vi "LOG_AppendEvent.vi"(8 "error in (no error)":errorcluster, 10 "Log Event":T1, 11 "String in":string) -> (0 "error out":errorcluster, 3 "String out":string)   [LabVIEW 2014]
uses:
  Controls/LOG_MessageQueue.ctl
  <userlib>/_OpenG.lib/string/string.llb/Trim Whitespace (String)__ogtk.vi
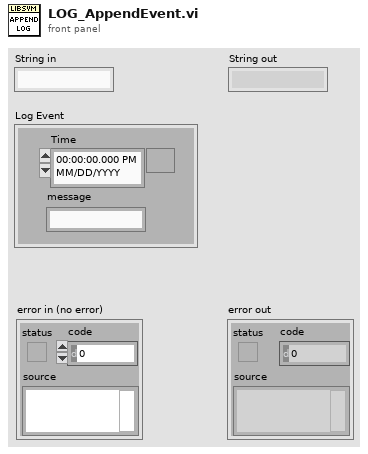
[diagram p1: front panel]
types:
  T1 = typedef "LOG_MessageQueue.ctl" = cluster{"Time":timestamp, "message":string}
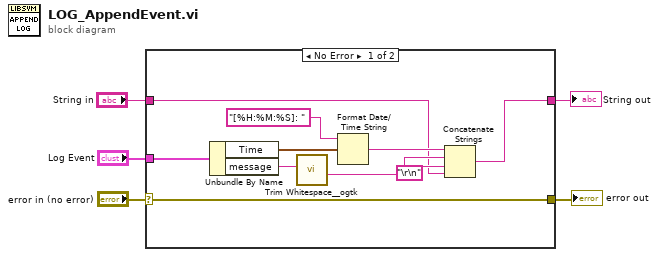
[diagram p0: block diagram]
diagram:
  n1 = case shown="No Error" "error in (no error)" {
    selector: "error in (no error)" -> [w6 w17]
    tunnel: [w6 w17] -> w5
    tunnel: [w9 w16] -> w3
    tunnel: "Log Event" -> [w8 _]
    tunnel: "String in" -> [w7 w16]
    frame No Error {
      n2 = Unbundle By Name(w8) -> ("Time"=w13:timestamp, "message"=w11:string)
      n3 = call-poly <userlib>:"Trim Whitespace__ogtk.vi"("String in"=w11) -> ("String out"=w12:string)  [unwired: 6 in]
      n4 = Format Date/Time String(time format string (%c)="[%H:%M:%S]: ", seconds (now)=w13) -> (date/time string=w15:string)  [unwired: 1 in]
      n5 = Concatenate Strings(w15, w12, "\r\n", w7) -> (w9:string)
    }
    frame Error {
    }
  }
  "error out" <- w5
  "String out" <- w3
